vi "Arduino_photo_resistance.vi"() -> ()   [LabVIEW 2013]
uses:
  <vilib>/Instr/_visa.llb/VISA Configure Serial Port (Instr).vi
panel:
  out "Light Sensor":dbl[](graph)
  out "Light Sensor":cluster{dbl, dbl}(graph)
  out "Resistance (Ohm)":dbl
  in  "stop":bool
  out "Intensity (a.u.)":dbl
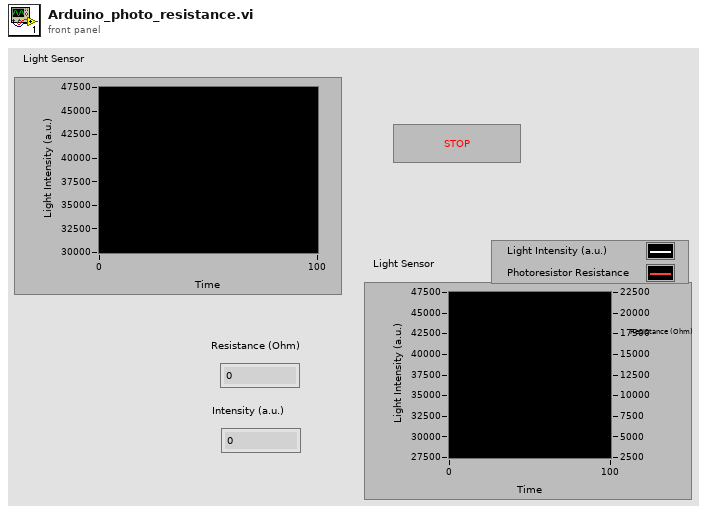
[diagram p1: front panel]
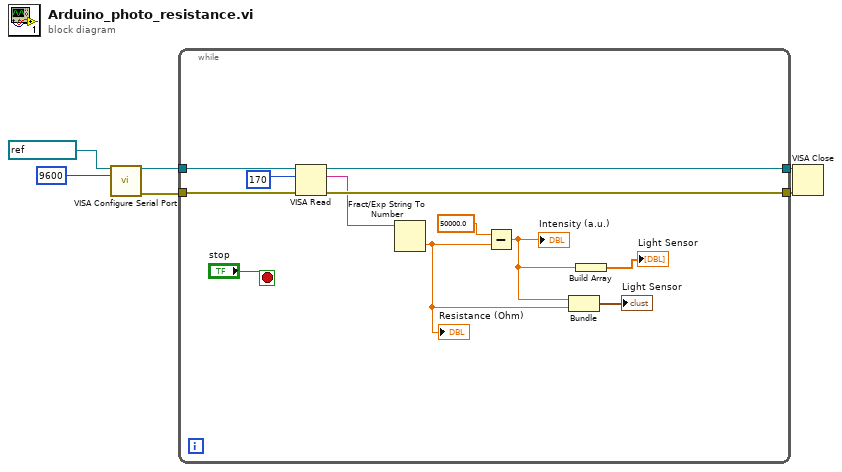
[diagram p0: block diagram]
diagram:
  n1 = call-poly "VISA Configure Serial Port"("VISA resource name"=refnum<visa-resource-name> "COM12", "baud rate (9600)"=u32 9600) -> ("VISA resource name out"=w3:refnum<visa-resource-name>, "error out"=w4:errorcluster)  [unwired: 12 in]
  n2 = while {
    tunnel: w3 -> [w14]
    tunnel: w4 -> [w13]
    tunnel: [w17] -> w6
    tunnel: [w16] -> w5
    stop <- "stop" stop-if-true
    n3 = VISA Read(VISA resource name=w14, byte count=u32 170, error in (no error)=w13) -> (VISA resource name out=w17:refnum<visa-resource-name>, read buffer=w12:string, error out=w16:errorcluster)  [unwired: 1 out]
    n4 = Fract/Exp String To Number(string=w12) -> (number=w10:dbl)  [unwired: 3 in, 1 out]
    "Resistance (Ohm)" <- w10
    n5 = Subtract(x=50000.0 ("y"), y=w10) -> (x-y=w8:dbl)
    "Intensity (a.u.)" <- w8
    n6 = Bundle(w8, w10) -> (→"Light Sensor":cluster{dbl, dbl})  [unwired: 1 in]
    n7 = Build Array(w8) -> (→"Light Sensor":dbl[])
  }
  n8 = VISA Close(VISA resource name=w6, error in (no error)=w5) -> ()  [unwired: 1 out]
